vi "gun_rt.vi"() -> ()   [LabVIEW 2011]
uses:
  gun_rt_slow_downstream_data.ctl
  gun_rt_fast_downstream_data.ctl
  gun_motor_state.ctl
  <vilib>/Platform/TimedLoop/XDataNode/timing_clust.ctl
  <vilib>/Platform/TimedLoop/XDataNode/nitl_modes.ctl
  <vilib>/Platform/TimedLoop/XDataNode/wakeup.ctl
  dashboard/dashboard_data_gun_fast.ctl
  gun_tracking_mode.ctl
  <vilib>/Rock Robotics/WPI/Joystick/WPI_JoystickDevRef.ctl
  <vilib>/Rock Robotics/WPI/Joystick/WPI_JoystickDeviceEnum.ctl
  signals/Signal.ctl
  gun_rt_slow_upstream_data.ctl
  idg_trust_t.ctl
  gun_rt_fast_upstream_data.ctl
  <vilib>/Platform/TimedLoop/XDataNode/XDataNode.xnode
  <vilib>/Platform/TimedLoop/XDataNode/XDNodeRunTimeDep.lvlib
panel:
  out "Waveform Chart 2":dbl(graph)
  out "Waveform Chart":cluster{"rpm raw":dbl, "Sensor Speed (rps)":dbl}(graph)
  in  "gun_rt_fast_downstream_data out":T1
  in  "gun_rt_slow_downstream_data out":T3
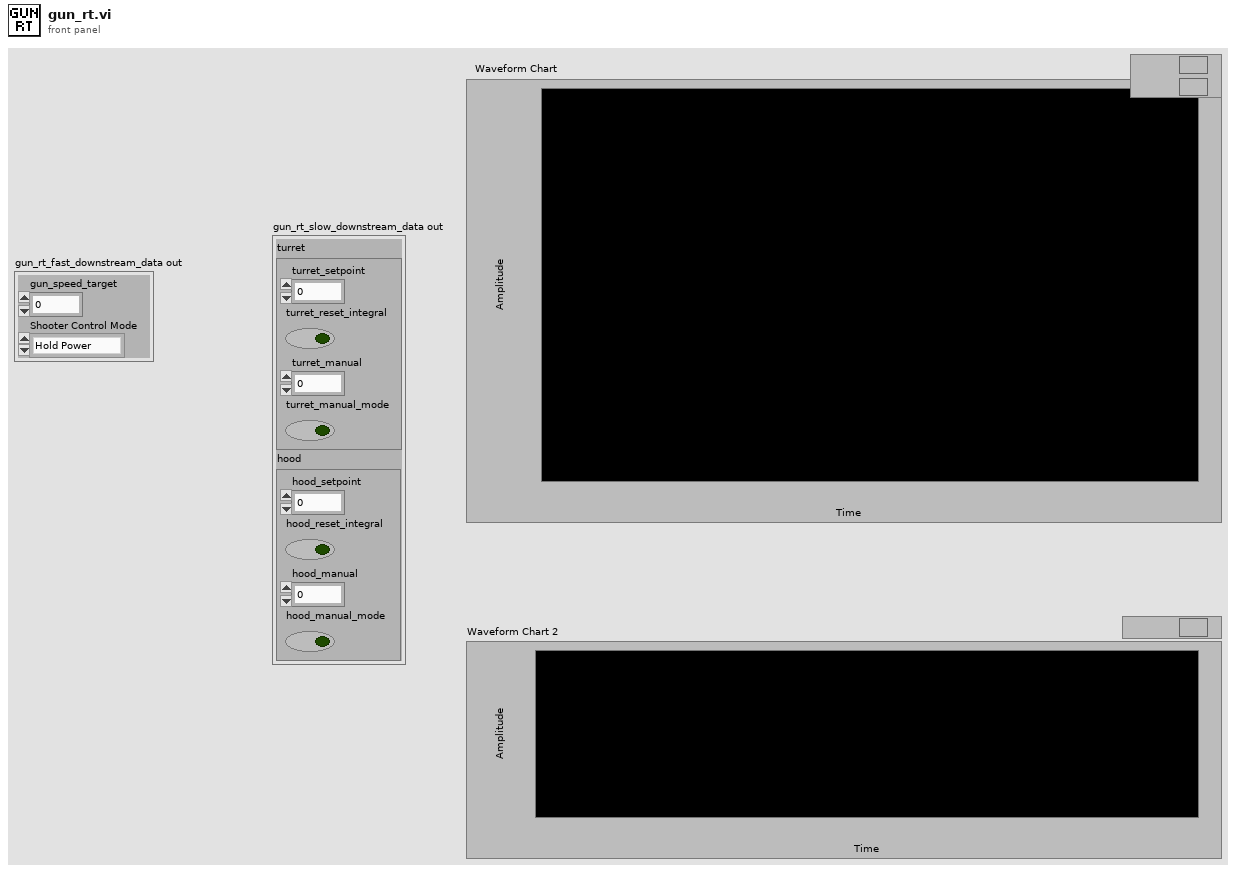
[diagram p1: front panel]
types:
  T1 = typedef "gun_rt_fast_downstream_data.ctl" = cluster{"gun_speed_target":dbl, "Shooter Control Mode":T2}
  T2 = typedef "gun_motor_state.ctl" = enum16{"Hold Power", "Hold Speed", "Hold Distance", "Stop"}
  T3 = typedef "gun_rt_slow_downstream_data.ctl" = cluster{"turret":cluster{"turret_setpoint":dbl, "turret_reset_integral":bool, "turret_manual":dbl, "turret_manual_mode":bool}, "hood":cluster{"hood_setpoint":dbl, "hood_reset_integral":bool, "hood_manual":dbl, "hood_manual_mode":bool}}
  T4 = typedef "dashboard_data_gun_fast.ctl" = cluster{"speed_setpoint":dbl, "speed_sensor":dbl, "gun_power":dbl, "gun_control_mode":T2, "gun_tracking_mode":T5}
  T5 = typedef "gun_tracking_mode.ctl" = enum16{"manual_aim", "auto_aim_camera", "preset_center_field", "preset_right_pocket", "preset_left_pocket", "align_center", "align_center_backwards", "auto_aim_key", "align_fold", "auton_custom", "preset_pass", "auto_aim_auton"}
  T6 = typedef "WPI_MotorControlDeviceRef.ctl" = cluster{"DeviceStatus":errorcluster, "Type":enum16{"PWM", "CAN"}, "PWM":cluster{"Digital Module":T7, "PWM Channel":T8, "DeadBand":T9}, "CAN":cluster{"Device Number":u8, "Control Mode":T10, "Semaphore":T11, "Max Vout":dbl}, "Invert":bool, "TransformRef":T12, "InvTransformRef":T12}
  T7 = typedef "FPGA_TypedefDigitalModule.ctl" = enum16{"Digital Module 1", "Digital Module 2"}
  T8 = typedef "FPGA_DIOPWMChannel.ctl" = enum8{"PWM 1", "PWM 2", "PWM 3", "PWM 4", "PWM 5", "PWM 6", "PWM 7", "PWM 8", "PWM 9", "PWM 10", "Invalid"}
  T9 = typedef "WPI_PWMDeadband.ctl" = cluster{"Name":string, "maxPositivePwm":i32, "minPositivePwm":i32, "centerPwm":i32, "maxNegativePwm":i32, "minNegativePwm":i32, "angularRange":u16}
  T10 = typedef "WPI_CANJaguar_ControlMode.ctl" = enum8{"Percent VBus", "Current", "Speed", "Position", "Voltage"}
  T11 = typedef "Semaphore RefNum" = refnum<k1>
  T12 = typedef "WPI_PWMTransform_ConPane.ctl" = refnum<vi>
  T13 = typedef "WPI_CounterDevRef.ctl" = cluster{"DevStatus":errorcluster, "CntIndex":T14}
  T14 = typedef "FPGA_CounterCtrSystemIndex.ctl" = enum8{"Ctr 0", "Ctr 1", "Ctr 2", "Ctr 3", "Ctr 4", "Ctr 5", "Ctr 6", "Ctr 7", "Invalid"}
  T15 = typedef "WPI_AnalogChannelDevRef.ctl" = cluster{"DevStatus":errorcluster, "Analog Module":T16, "Analog Channel":T17}
  T16 = typedef "FPGA_TypedefAnalogModule.ctl" = enum16{"Analog Module 1", "Analog Module 2"}
  T17 = typedef "FPGA_AIChannel.ctl" = enum8{"AI 1", "AI 2", "AI 3", "AI 4", "AI 5", "AI 6", "AI 7", "AI 8", "Invalid"}
  T18 = enum16{"push_data", "write_joe_johnson", "write_roller", "write_drivetrain", "write_gun_fast", "write_gun_slow"}
  T19 = typedef "WPI_JoystickDevRef.ctl" = cluster{"Device":T20}
  T20 = typedef "WPI_JoystickDeviceEnum.ctl" = enum16{"USB 1", "USB 2", "USB 3", "USB 4", "Kinect 1", "Kinect 2"}
  T21 = typedef "Signal.ctl" = enum16{"SIGFIRE", "SIGSTOPSCRIPT", "SIGSTARTGUN", "SIGSTOPGUN", "SIGDISABLED", "SIGENABLED", "SIGUDPTIMEOUT", "SIGNEWVISION_REMOTE", "SIGNEWVISION_LOCAL", "SIGSHOTFIRED", "SIGDOTRACK", "SIGDONTTRACK"}
  T22 = typedef "gun_rt_slow_upstream_data.ctl" = cluster{"turret":cluster{"turret_analog":dbl, "turret_angle":dbl, "turret_motor":dbl, "turret_idg_state":T23}, "hood":cluster{"hood_analog":dbl, "hood_angle":dbl, "hood_motor":dbl, "hood_idg_state":T23}}
  T23 = typedef "idg_trust_t.ctl" = enum16{"fault_move", "fault_high", "fault_low", "out_high", "out_low", "trust"}
  T24 = typedef "gun_const_t.ctl" = cluster{"gun":cluster{"num_lines":dbl, "gain_kp1":dbl, "gain_kp2":dbl, "gain_ki":dbl, "gain_kd":dbl}, "turret":cluster{"center_ana":dbl, "volts_per_180":dbl, "man_scale":dbl, "turret_idg":T25, "turret_pid":T26, "turret_invert":bool, "turret_low_power":dbl}, "tracking":cluster{"velocity_lead_gain":dbl, "velocity_rotation_gain":dbl}, "hood":cluster{"hood_idg":T25, "hood_pid":T26, "hood_scale":T27, "hood_invert":bool}}
  T25 = typedef "gun_idg_const.ctl" = cluster{"low_fault_ana":dbl, "high_fault_ana":dbl, "min_ana":dbl, "max_ana":dbl, "movement_thresh":dbl, "movement_time":dbl}
  T26 = typedef "gain_const.ctl" = cluster{"kP":dbl, "kI":dbl, "kD":dbl}
  T27 = typedef "scale_const.ctl" = cluster{"min_ana":dbl, "min_units":dbl, "max_ana":dbl, "max_units":dbl}
  T28 = cluster{"axis 1 (x)":dbl, "axis 2 (y)":dbl, "axis 3 (throttle)":dbl, "axis 4":dbl, "axis 5":dbl, "axis 6":dbl}
  T29 = typedef "XDNodeRunTimeDep.lvlib/timing_clust.ctl" = cluster{"Expected End [f-1]":u64, "Actual End [f-1]":u64, "Finished Late? [f-1]":bool, "Expected End [i-1]":u64, "Actual End [i-1]":u64, "Finished Late? [i-1]":bool, "Expected Start [i]":u64, "Actual Start [i]":u64, "Expected Start [f]":u64, "Actual Start [f]":u64, "Source Name":string, "Structure Name":string, "Period":i64, "Deadline":i64, "Offset":i64, "Start":i64, "Priority":i32, "Timeout":i32, "Mode":T30, "Wakeup Reason":T31, "Error":errorcluster, "Source Type":string, "Secondary Source Type":string, "Global End Time":u64, "Global Start Time":u64, "Frame Duration":u64, "Iteration Duration":u64, "Assigned CPU":i32, "I/O Scan Engine Mode":u32}
  T30 = typedef "XDNodeRunTimeDep.lvlib/nitl_modes.ctl" = enum32{"No Change", "Process missed periods, maintain original phase", "Discard missed periods, maintain original phase", "Process missed periods, ignore original phase", "Discard missed periods, ignore original phase"}
  T31 = typedef "XDNodeRunTimeDep.lvlib/wakeup.ctl" = enum32{"Normal", "Aborted", "Asynchronous wakeup", "Timing source error", "Timed loop error", "Timeout"}
  T32 = typedef "gun_rt_fast_upstream_data.ctl" = cluster{"gun_sensor_speed":dbl, "gun_motor_output":dbl}
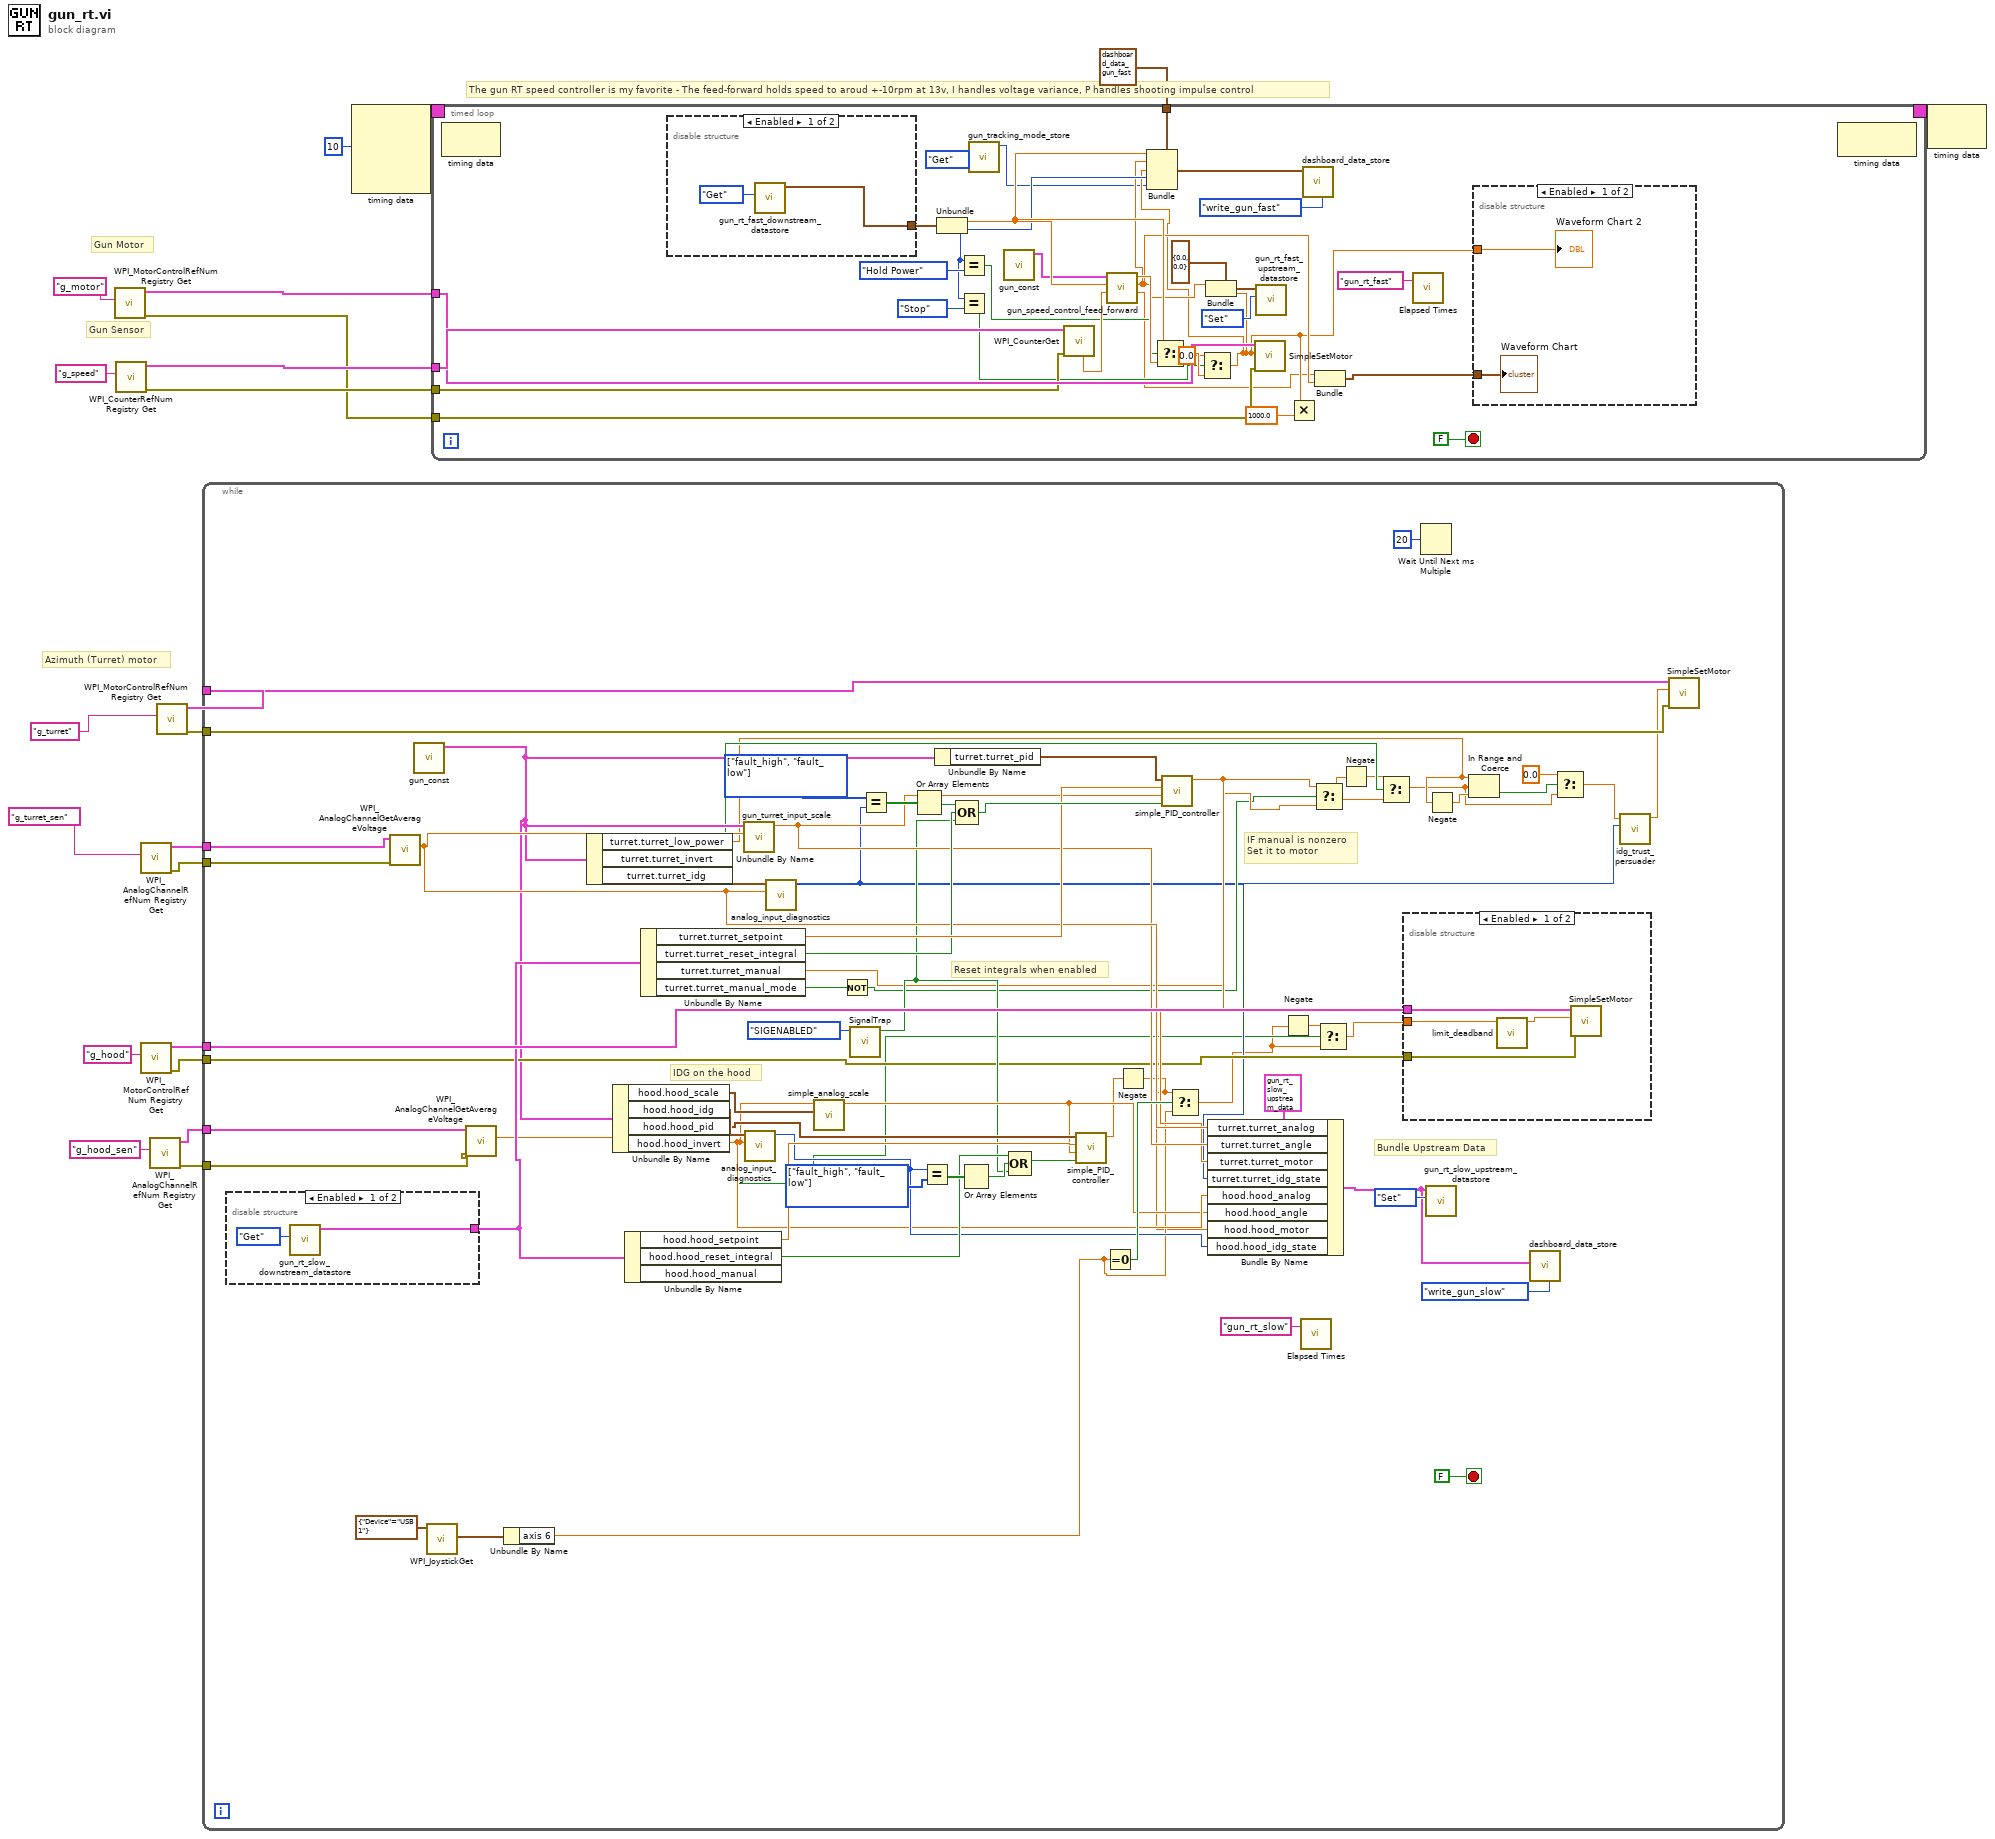
[diagram p0: block diagram]
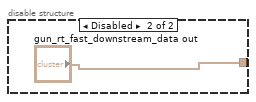
[diagram p3: hidden frame]
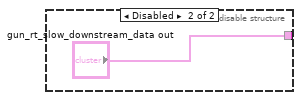
[diagram p5: hidden frame]
diagram:
  # "The gun RT speed controller is my favorite - The feed-forward holds speed to aroud +-10rpm at 13v, I handles voltage variance, P handles shooting impulse control"
  # "Gun Sensor"
  # "Gun Motor"
  # "Azimuth (Turret) motor"
  n1 = call <vilib>:"WPI_MotorControlRefNum Registry Get.vi"("refnum name"="g_motor") -> ("error out"=w5:errorcluster, "MotorControlDevRef"=w9:T6)  [unwired: 9 in]
  n2 = call <vilib>:"WPI_CounterRefNum Registry Get.vi"("refnum name"="g_speed") -> ("error out"=w6:errorcluster, "CounterDevRef"=w10:T13)  [unwired: 9 in]
  n3 = call <vilib>:"WPI_AnalogChannelRefNum Registry Get.vi"("refnum name"="g_turret_sen") -> ("error out"=w14:errorcluster, "AIDeviceRef"=w20:T15)  [unwired: 9 in]
  n4 = call <vilib>:"WPI_MotorControlRefNum Registry Get.vi"("refnum name"="g_hood") -> ("error out"=w11:errorcluster, "MotorControlDevRef"=w16:T6)  [unwired: 9 in]
  n5 = call <vilib>:"WPI_AnalogChannelRefNum Registry Get.vi"("refnum name"="g_hood_sen") -> ("error out"=w13:errorcluster, "AIDeviceRef"=w15:T15)  [unwired: 9 in]
  n6 = call <vilib>:"WPI_MotorControlRefNum Registry Get.vi"("refnum name"="g_turret") -> ("error out"=w12:errorcluster, "MotorControlDevRef"=w19:T6)  [unwired: 9 in]
  n7 = while {
    tunnel: w20 -> [w87]
    tunnel: w19 -> [w86]
    tunnel: w16 -> [w85]
    tunnel: w15 -> [w84]
    tunnel: w14 -> [w53]
    tunnel: w13 -> [w52]
    tunnel: w12 -> [w51]
    tunnel: w11 -> [w50]
    stop <- FALSE stop-if-true
    w75 = T23[] [enum."fault_high", enum."fault_low"] items=["fault_move", "fault_high", "fault_low", "out_high", "out_low", "trust"]
    w80 = T23[] [enum."fault_high", enum."fault_low"] items=["fault_move", "fault_high", "fault_low", "out_high", "out_low", "trust"]
    # "Bundle Upstream Data"
    # "IF manual is nonzero\nSet it to motor"
    # "Reset integrals when enabled"
    # "IDG on the hood"
    n8 = disable-structure shown="Enabled" {
      disable-tunnel: [w93 "gun_rt_slow_downstream_data out"] -> w68
      frame Enabled {
        n9 = call "gun_rt_slow_downstream_datastore.vi"("data_store_mode"=enum16{"Set", "Get"}."Get") -> ("gun_rt_slow_downstream_data out"=w93:T3)  [unwired: 10 in]
      }
      frame Disabled {
      }
    }
    n10 = call <vilib>:"WPI_AnalogChannelGetAverageVoltage.vi"("error in (no error)"=w53, "AIDeviceRef"=w87) -> ("Voltage"=w61:dbl)  [unwired: 7 in, 2 out]
    n11 = call "gun_const.vi"() -> ("Data Out"=w43:T24)  [unwired: 11 in]
    n12 = call <vilib>:"WPI_JoystickGet.vi"("JoystickDevRef"=T19 {"Device"=enum."USB 1"}) -> ("Axes"=w47:T28)  [unwired: 4 in, 2 out]
    n13 = call <vilib>:"WPI_AnalogChannelGetAverageVoltage.vi"("error in (no error)"=w52, "AIDeviceRef"=w84) -> ("Voltage"=w58:dbl)  [unwired: 7 in, 2 out]
    n14 = Unbundle By Name(w47) -> ("axis 6"=w46:dbl)
    n15 = Unbundle By Name(w43) -> ("turret.turret_low_power"=w38:dbl, "turret.turret_invert"=w42:bool, "turret.turret_idg"=w79:T25)
    n16 = Unbundle By Name(w43) -> ("hood.hood_scale"=w76:T27, "hood.hood_idg"=w78:T25, "hood.hood_pid"=w72:T26, "hood.hood_invert"=w28:bool)
    n17 = Unbundle By Name(w68) -> ("hood.hood_setpoint"=w67:dbl, "hood.hood_reset_integral"=w66:bool)  [unwired: 1 out]
    n18 = Unbundle By Name(w68) -> ("turret.turret_setpoint"=w70:dbl, "turret.turret_reset_integral"=w69:bool, "turret.turret_manual"=w34:dbl, "turret.turret_manual_mode"=w33:bool)
    n19 = call "gun_turret_input_scale.vi"("Voltage"=w61, "Gun Const"=w43) -> ("Angle"=w60:dbl)  [unwired: 9 in]
    n20 = call "analog_input_diagnostics.vi"("Voltage"=w58, "IDG Const"=w78) -> ("IDG State"=w62:T23)  [unwired: 7 in, 2 out]
    n21 = call "analog_input_diagnostics.vi"("Voltage"=w61, "IDG Const"=w79) -> ("IDG State"=w29:T23)  [unwired: 7 in, 2 out]
    n22 = call "simple_analog_scale.vi"("Scale Const"=w76, "Analog"=w58) -> ("Units"=w57:dbl)  [unwired: 9 in]
    n23 = Not(x=w33) -> (.not. x?=w32:bool)
    n24 = call "SignalTrap.vi"("Signal"=Signal."SIGENABLED") -> ("Trapped Signal"=w55:bool)  [unwired: 10 in]
    n25 = Equal?(x=w80, y=w29) -> (x = y?=w81:bool[])
    n26 = Or Array Elements(Boolean array=w81) -> (logical OR=w82:bool)
    n27 = Equal?(x=w62, y=w75) -> (x = y?=w74:bool[])
    n28 = Unbundle By Name(w43) -> ("turret.turret_pid"=w77:T26)
    n29 = Compound Arithmetic op=OR(w82, w69, w55) -> (w83:bool)
    n30 = Or Array Elements(Boolean array=w74) -> (logical OR=w73:bool)
    n31 = Compound Arithmetic op=OR(w66, w73, w55) -> (w71:bool)
    n32 = call "simple_PID_controller.vi"("Reset Integral"=w71, "Sensor"=w57, "Setpoint"=w67, "PID Const"=w72) -> ("Motor Power"=w45:dbl)  [unwired: 7 in]
    n33 = Equal To 0?(x=w46) -> (x = 0?=w65:bool)
    n34 = Negate(x=w45) -> (-x=w44:dbl)
    n35 = call "simple_PID_controller.vi"("Reset Integral"=w83, "Sensor"=w60, "Setpoint"=w70, "PID Const"=w77) -> ("Motor Power"=w59:dbl)  [unwired: 7 in]
    n36 = Select(t=w44, s=w65, f=w46) -> (s? t:f=w25:dbl)
    n37 = Bundle By Name(cluster=T22 {"turret"={"turret_analog"=0.0, "turret_angle"=0.0, "turret_motor"=0.0, "turret_idg_state"=enum."fault_high"}, "hood"={"hood_analog"=0.0, "hood_angle"=0.0, "hood_motor"=0.0, "hood_idg_state"=enum."fault_high"}} ("gun_rt_slow_upstream_data"), "turret.turret_analog"=w61, "turret.turret_angle"=w60, "turret.turret_motor"=w59, "turret.turret_idg_state"=w29, "hood.hood_analog"=w58, "hood.hood_angle"=w57, "hood.hood_motor"=w44, "hood.hood_idg_state"=w62) -> (w23:T22)
    n38 = Negate(x=w25) -> (-x=w26:dbl)
    n39 = call "Elapsed Times.vi"("Call Name"="gun_rt_slow") -> ()  [unwired: 2 in, 1 out]
    n40 = Select(t=w59, s=w32, f=w34) -> (s? t:f=w40:dbl)
    n41 = Select(t=w26, s=w28, f=w25) -> (s? t:f=w27:dbl)
    n42 = Negate(x=w40) -> (-x=w41:dbl)
    n43 = Select(t=w41, s=w42, f=w40) -> (s? t:f=w37:dbl)
    n44 = disable-structure shown="Enabled" {
      disable-tunnel: w85 -> [w92 _]
      disable-tunnel: w50 -> [w91 _]
      disable-tunnel: w27 -> [w89 _]
      frame Enabled {
        n45 = call "limit_deadband.vi"("Val"=w89) -> ("Val Out"=w90:dbl)  [unwired: 10 in]
        n46 = call "SimpleSetMotor.vi"("error in (no error)"=w91, "Output"=w90, "MotorControlDevRef"=w92) -> ()  [unwired: 7 in, 2 out]
      }
      frame Disabled {
      }
    }
    n47 = Wait Until Next ms Multiple(millisecond multiple=u32 20) -> ()  [unwired: 1 out]
    n48 = call "gun_rt_slow_upstream_datastore.vi"("data_store_mode"=enum16{"Set", "Get"}."Set", "gun_rt_slow_upstream_data"=w23) -> ()  [unwired: 9 in, 1 out]
    n49 = Negate(x=w38) -> (-x=w39:dbl)
    n50 = In Range and Coerce(upper limit=w38, x=w37, lower limit=w39) -> (In Range?=w36:bool)  [unwired: 1 out]
    n51 = call "dashboard_data_store.vi"("mode"=T18."write_gun_slow", "gun_slow"=w23) -> ()  [unwired: 10 in]
    n52 = Select(t=0.0, s=w36, f=w37) -> (s? t:f=w31:dbl)
    n53 = call "idg_trust_persuader.vi"("Input Diagnostic State"=w29, "output"=w31) -> ("output out"=w30:dbl)  [unwired: 9 in]
    n54 = call "SimpleSetMotor.vi"("error in (no error)"=w51, "Output"=w30, "MotorControlDevRef"=w86) -> ()  [unwired: 7 in, 2 out]
  }
  n55 = node-c288(i64 10 ("Period")) -> (w4:T29)  [unwired: 3 in]
  n56 = timed-loop {
    tunnel: w10 -> [w126]
    tunnel: w9 -> [w125]
    tunnel: w6 -> [w118]
    tunnel: w5 -> [w117]
    timing: w4 -> [_]
    timing-out: [_] -> w3
    tunnel: T4 {"speed_setpoint"=0.0, "speed_sensor"=0.0, "gun_power"=0.0, "gun_control_mode"=enum."Hold Power", "gun_tracking_mode"=enum."manual_aim"} ("gun_fast") -> [w109]
    stop <- FALSE stop-if-true
    n57 = node-c288() -> ()  [unwired: 1 in, 1 out]
    n58 = disable-structure shown="Enabled" {
      disable-tunnel: [w131 "gun_rt_fast_downstream_data out"] -> w123
      frame Enabled {
        n59 = call "gun_rt_fast_downstream_datastore.vi"("data_store_mode"=enum16{"Set", "Get"}."Get") -> ("gun_rt_fast_downstream_data out"=w131:T1)  [unwired: 10 in]
      }
      frame Disabled {
      }
    }
    n60 = Unbundle(w123) -> ("gun_speed_target"=w108:dbl, "Shooter Control Mode"=w107:T2)
    n61 = Equal?(x=w107, y=gun_motor_state."Hold Power") -> (x = y?=w114:bool)
    n62 = Equal?(x=w107, y=gun_motor_state."Stop") -> (x = y?=w111:bool)
    n63 = call "gun_tracking_mode_store.vi"("data_store_mode"=enum16{"Set", "Get"}."Get") -> ("gun tracking mode"=w98:T5)  [unwired: 10 in]
    n64 = call "gun_const.vi"() -> ("Data Out"=w104:T24)  [unwired: 11 in]
    n65 = call <vilib>:"WPI_CounterGet.vi"("error in (no error)"=w118, "CounterDevRef in"=w126) -> ("Period (sec)"=w124:dbl)  [unwired: 4 in, 5 out]
    n66 = call "gun_speed_control_feed_forward.vi"("Period (sec)"=w124, "Speed (rps)"=w108, "Gun Const"=w104) -> ("rpm raw"=w100:dbl, "Sensor Speed (rps)"=w106:dbl, "Output"=w115:dbl)  [unwired: 6 in]
    n67 = Select(t=w108, s=w114, f=w115) -> (s? t:f=w112:dbl)
    n68 = Select(t=0.0, s=w111, f=w112) -> (s? t:f=w102:dbl)
    n69 = Bundle(cluster=w109, "speed_setpoint"=w108, "speed_sensor"=w106, "gun_power"=w102, "gun_control_mode"=w107, "gun_tracking_mode"=w98) -> (w97:T4)
    n70 = Bundle(cluster=T32 {"gun_sensor_speed"=0.0, "gun_motor_output"=0.0} ("gun_rt_fast_upstream_data"), "gun_sensor_speed"=w106, "gun_motor_output"=w102) -> (w120:T32)
    n71 = call "SimpleSetMotor.vi"("error in (no error)"=w117, "Output"=w102, "MotorControlDevRef"=w125) -> ()  [unwired: 7 in, 2 out]
    n72 = call "gun_rt_fast_upstream_datastore.vi"("data_store_mode"=enum16{"Set", "Get"}."Set", "gun_rt_fast_upstream_data"=w120) -> ()  [unwired: 9 in, 1 out]
    n73 = Multiply(x=w102, y=1000.0) -> ()  [unwired: 1 out]
    n74 = call "dashboard_data_store.vi"("mode"=T18."write_gun_fast", "gun_fast"=w97) -> ()  [unwired: 10 in]
    n75 = Bundle("rpm raw"=w100, "Sensor Speed (rps)"=w106) -> (w101:cluster{"rpm raw":dbl, "Sensor Speed (rps)":dbl})  [unwired: 1 in]
    n76 = call "Elapsed Times.vi"("Call Name"="gun_rt_fast") -> ()  [unwired: 2 in, 1 out]
    n77 = disable-structure shown="Enabled" {
      disable-tunnel: w102 -> [w128 _]
      disable-tunnel: w101 -> [w127 _]
      frame Enabled {
        "Waveform Chart" <- w127
        "Waveform Chart 2" <- w128
      }
      frame Disabled {
      }
    }
    n78 = node-c288() -> ()  [unwired: 1 in, 1 out]
  }
  n79 = node-c288(w3) -> ()  [unwired: 1 out]
